vi "Hz to RPM.vi"(11 "Hz":dbl[unit]) -> (3 "speed out (rpm)":dbl)   [LabVIEW 2019]
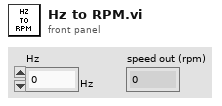
[diagram p1: front panel]
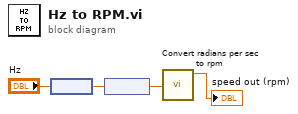
[diagram p0: block diagram]
diagram:
  n1 = node("Hz") -> (w1:dbl)
  n2 = node(w1) -> (w3:dbl[unit])
  n3 = call "Convert radians per sec to rpm.vi"("speed in"=w3) -> ("speed out (rpm)"=→"speed out (rpm)":dbl)  [unwired: 10 in]
